vi "Send Data.vi"(8 "error in (no error)":errorcluster, 11 "ValveControlModule in":refnum<class "ValveControlModule.lvclass">) -> (0 "error out":errorcluster, 3 "ValveControlModule out":refnum<class "ValveControlModule.lvclass">)   [LabVIEW 2020, in "VolatusControl.lvlib" / "ValveControlModule.lvclass"]
uses:
  ValveControlModule.lvclass
  ValveControlModule.lvclass/ValveControlModule.ctl
  VolatusData/VolatusData.lvlib
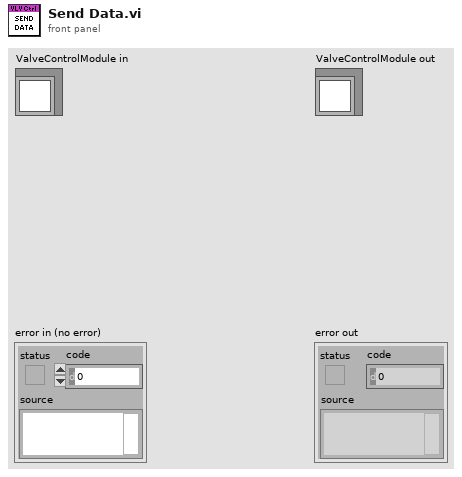
[diagram p1: front panel]
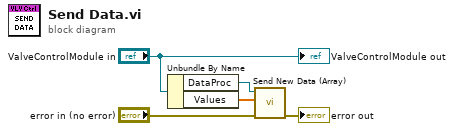
[diagram p0: block diagram]
diagram:
  n1 = Unbundle By Name("ValveControlModule in") -> ("DataProc"=w4:refnum<class "MessageQ.lvclass">, "Values"=w3:dbl[])
  n2 = call "Send New Data (Array).vi"("error in (no error)"="error in (no error)", "Data"=w3, "MessageQ"=w4) -> ("error out"=→"error out":errorcluster)  [unwired: 8 in]
  "ValveControlModule out" <- "ValveControlModule in"
